vi "Kinesis-Teste-Vector-1.vi"() -> ()   [LabVIEW 2014]
doc: "André Romero - 2017\nandretec@ifsc.usp.br"
uses:
  Basic-VIs/motorsGlobalVar.vi
  <vilib>/Instr/_visa.llb/VISA Configure Serial Port (Instr).vi
  C:/user-Lab/AndreTec/GITs/andretec/Thorlabs-Vector-Move/kinesisTec/Kinesis/Thorlabs.MotionControl.TCube.DCServoCLI.dll
  kinesisTec/Kinesis/Thorlabs.MotionControl.TCube.DCServoCLI.dll
  C:/user-Lab/AndreTec/GITs/andretec/Thorlabs-Vector-Move/kinesisTec/Kinesis/Thorlabs.MotionControl.GenericMotorCLI.dll
  kinesisTec/Kinesis/Thorlabs.MotionControl.GenericMotorCLI.dll
  C:/user-Lab/AndreTec/GITs/andretec/Thorlabs-Vector-Move/kinesisTec/Kinesis/Thorlabs.MotionControl.Controls.dll
  kinesisTec/Kinesis/Thorlabs.MotionControl.Controls.dll
panel:
  out "IsAtHWLimit 2":bool
  out "IsAtHWLimit":bool
  in  "stop":bool
  in  "Adjust Motors":bool
  out "Process time":string="0:00:50"
  out "Progress %":dbl(slide) scale=0.0..100.0
  out "XY Graph":cluster{"Graph X":dbl[], "Graph Y":dbl[]}(graph)
  in  "Swap XY":bool
  out "stop cronometro":bool=TRUE
  in  "Stop Button":bool
  in  "Graph Y":dbl[](array[numeric])=[0.0, 0.0, 6.6674440298507465, 6.6674440298507465, 6.6674440298507465, 6.6674440298507465, 6.6674440298507465, 6.6674440298507465, 6.6674440298507465, 6.6674440298507465, 6.6674440298507465, 6.6674440298507465, 6.6674440298507465, 6.6674440298507465, 6.6674440298507465, 6.6674440298507465, 6.6674440298507465, 6.6674440298507465, 6.6674440298507465, 6.6674440298507465, 6.6674440298507465, 6.6674440298507465, 6.6674440298507465, 6.6674440298507465, 6.6674440298507465, 6.6674440298507465, 6.6674440298507465, 6.6674440298507465, 6.6674440298507465, 6.6674440298507465, 6.6674440298507465, 6.6674440298507465, 6.6674440298507465, 6.6674440298507465, 6.6674440298507465, 6.6674440298507465, 6.6674440298507465, 6.6674440298507465, 6.6674440298507465, 6.6674440298507465, 6.6674440298507465, 6.6674440298507465, 6.6674440298507465, 6.673128498134329, 6.673128498134329, 6.673128498134329, 6.673128498134329, 6.673128498134329, 6.687354244402985, 6.687354244402985, 6.687354244402985, 6.687354244402985, 6.687354244402985, 6.692543143656716, 6.692543143656716, 6.692543143656716, 6.692543143656716, 6.692543143656716, 6.692543143656716, 6.692543143656716, 6.692543143656716, 6.692543143656716, 6.692543143656716, 6.692543143656716, 6.692543143656716, 6.691522854477612, 6.691522854477612, 6.691522854477612, 6.691522854477612, 6.691522854477612, 6.680183069029851, 6.680183069029851, 6.680183069029851, 6.680183069029851, 6.680183069029851, 6.658640391791045, 6.658640391791045, 6.658640391791045, 6.658640391791045, 6.658640391791045, 6.644793610074627, 6.644793610074627, 6.644793610074627, 6.644793610074627, 6.644793610074627, 6.642490671641791, 6.642490671641791, 6.642490671641791, 6.642490671641791, 6.642490671641791, 6.642490671641791, 6.642490671641791, 6.642490671641791, 6.642490671641791, 6.642490671641791, 6.642490671641791, 6.642490671641791, 6.642490671641791, 6.642490671641791, 6.642490671641791, 6.647825326492537, 6.647825326492537, 6.647825326492537, 6.647825326492537, 6.647825326492537, 6.66543260261194, 6.66543260261194, 6.66543260261194, 6.66543260261194, 6.66543260261194, 6.685226212686567, 6.685226212686567, 6.685226212686567, 6.685226212686567, 6.685226212686567, 6.692484841417911, 6.692484841417911, 6.692484841417911, 6.692484841417911, 6.692484841417911, 6.692543143656716, 6.692543143656716, 6.692543143656716, 6.692543143656716, 6.692543143656716, 6.692543143656716, 6.692543143656716, 6.691464552238806, 6.691464552238806, 6.691464552238806, 6.691464552238806, 6.691464552238806, 6.679833255597015, 6.679833255597015, 6.679833255597015, 6.679833255597015, 6.679833255597015, 6.658057369402985, 6.658057369402985, 6.658057369402985, 6.658057369402985, 6.658057369402985, 6.644647854477612, 6.644647854477612, 6.644647854477612, 6.644647854477612, 6.644647854477612, 6.642548973880597, 6.642548973880597, 6.642548973880597, 6.642548973880597, 6.642548973880597, 6.642519822761194, 6.642519822761194, 6.642519822761194, 6.642519822761194, 6.642519822761194, 6.642519822761194, 6.642519822761194, 6.642519822761194, 6.643569263059701, 6.643569263059701, 6.643569263059701, 6.643569263059701, 6.643569263059701, 6.655521222014926, 6.655521222014926, 6.655521222014926, 6.655521222014926, 6.655521222014926, 6.677180503731344, 6.677180503731344, 6.677180503731344, 6.677180503731344, 6.677180503731344, 6.690531716417911, 6.690531716417911, 6.690531716417911, 6.690531716417911, 6.690531716417911, 6.692572294776119, 6.692572294776119, 6.692572294776119, 6.692572294776119, 6.692572294776119, 6.692572294776119, 6.692572294776119, 6.692572294776119, 6.692572294776119, 6.692572294776119, 6.692572294776119, 6.692572294776119, 6.691522854477612, 6.691522854477612, 6.691522854477612, 6.691522854477612, 6.691522854477612, 6.680008162313433, 6.680008162313433, 6.680008162313433, 6.680008162313433, 6.680008162313433, 6.668668376865671, 6.668668376865671, 6.668668376865671, 6.668668376865671, 6.668668376865671, 6.667502332089552, 6.667502332089552, 6.667502332089552, 6.667502332089552, 6.667502332089552, 6.667502332089552, 6.667502332089552, 6.667502332089552, 6.667502332089552, 6.667502332089552, 6.667502332089552, 6.667502332089552, 6.667531483208955, 6.667531483208955, 6.667531483208955, 6.667531483208955, 6.667531483208955, 6.667531483208955, 6.667531483208955, 6.667531483208955, 6.667531483208955, 6.667531483208955, 6.667531483208955, 6.667531483208955, 6.667531483208955, 6.667531483208955, 6.667531483208955, 6.667531483208955, 6.667531483208955, 6.667531483208955, 6.667531483208955, 6.667531483208955, 6.667531483208955, 6.667531483208955, 6.667531483208955, 6.667531483208955, 6.667531483208955, 6.667531483208955, 6.667531483208955, 6.667531483208955, 6.667531483208955, 6.667531483208955, 6.667531483208955, 6.667531483208955, 6.667531483208955, 6.667531483208955, 6.667531483208955, 6.667531483208955, 6.667531483208955, 6.6663945895522385, 6.6663945895522385, 6.6663945895522385, 6.6663945895522385, 6.6663945895522385, 6.662051072761194, 6.662051072761194, 6.662051072761194, 6.662051072761194, 6.662051072761194, 6.644035680970149, 6.644035680970149, 6.644035680970149, 6.644035680970149, 6.644035680970149, 6.606430736940299, 6.606430736940299, 6.606430736940299, 6.606430736940299, 6.606430736940299, 6.593924906716418, 6.593924906716418, 6.593924906716418, 6.593924906716418, 6.593924906716418, 6.574539412313433, 6.574539412313433, 6.574539412313433, 6.574539412313433, 6.574539412313433, 6.567484841417911, 6.567484841417911, 6.567484841417911, 6.567484841417911, 6.567484841417911, 6.567484841417911, 6.567484841417911, 6.567484841417911, 6.567484841417911, 6.567484841417911, 6.567484841417911, 6.567513992537314, 6.567513992537314, 6.567513992537314, 6.567513992537314, 6.567513992537314, 6.567513992537314, 6.567513992537314, 6.567513992537314, 6.567513992537314, 6.567513992537314, 6.567543143656716, 6.567543143656716, 6.567543143656716, 6.567543143656716, 6.567543143656716, 6.567543143656716, 6.567543143656716, 6.567543143656716, 6.567543143656716, 6.567543143656716, 6.567543143656716, 6.567543143656716, 6.567543143656716, 6.567543143656716, 6.567543143656716, 6.567543143656716, 6.567543143656716, 6.567543143656716, 6.567543143656716, 6.567543143656716, 6.567543143656716, 6.567543143656716, 6.567543143656716, 6.567543143656716, 6.567543143656716, 6.567543143656716, 6.567543143656716, 6.567543143656716, 6.567543143656716, 6.567543143656716, 6.567543143656716, 6.567543143656716, 6.567543143656716, 6.567543143656716, 6.567543143656716, 6.567543143656716, 6.567543143656716, 6.567543143656716, 6.567543143656716, 6.567543143656716, 6.567543143656716, 6.567543143656716, 6.567543143656716, 6.567543143656716, 6.567543143656716, 6.567543143656716, 6.567543143656716, 6.567543143656716, 6.567543143656716, 6.567543143656716, 6.567543143656716, 6.567543143656716, 6.567543143656716, 6.567543143656716, 6.5667852145522385, 6.5667852145522385, 6.5667852145522385, 6.5667852145522385, 6.5667852145522385, 6.555299673507463, 6.555299673507463, 6.555299673507463, 6.555299673507463, 6.555299673507463, 6.533523787313433, 6.533523787313433, 6.533523787313433, 6.533523787313433, 6.533523787313433, 6.525186567164179, 6.525186567164179, 6.525186567164179, 6.525186567164179, 6.525186567164179, 6.517490671641791, 6.517490671641791, 6.517490671641791, 6.517490671641791, 6.517490671641791, 6.517490671641791, 6.517490671641791, 6.517490671641791, 6.517490671641791, 6.517490671641791, 6.517519822761194, 6.517519822761194, 6.517519822761194, 6.517519822761194, 6.517519822761194, 6.517519822761194, 6.517519822761194, 6.517519822761194, 6.517519822761194, 6.517519822761194, 6.517548973880597, 6.517548973880597, 6.517548973880597, 6.517548973880597, 6.517548973880597, 6.517548973880597, 6.517548973880597, 6.517548973880597, 6.517548973880597, 6.517548973880597, 6.517548973880597, 6.517548973880597, 6.517548973880597, 6.517548973880597, 6.517548973880597, 6.517548973880597, 6.517548973880597, 6.517548973880597, 6.517548973880597, 6.517548973880597, 6.517548973880597, 6.517548973880597, 6.517548973880597, 6.517548973880597, 6.517548973880597, 6.517548973880597, 6.517548973880597, 6.517548973880597, 6.517548973880597, 6.517548973880597, 6.517548973880597, 6.517548973880597, 6.517548973880597, 6.517548973880597, 6.517548973880597, 6.517548973880597, 6.517548973880597, 6.517548973880597, 6.517548973880597, 6.517548973880597, 6.517548973880597, 6.517548973880597, 6.517548973880597, 6.517548973880597, 6.517548973880597, 6.517548973880597, 6.517548973880597, 6.517548973880597, 6.517548973880597, 6.517548973880597, 6.517548973880597, 6.517548973880597, 6.517548973880597, 6.517548973880597, 6.517548973880597, 6.517548973880597, 6.517548973880597, 6.517548973880597, 6.517548973880597, 6.517548973880597, 6.516674440298507, 6.516674440298507, 6.516674440298507, 6.516674440298507, 6.516674440298507, 6.504897388059701, 6.504897388059701, 6.504897388059701, 6.504897388059701, 6.504897388059701, 6.481926305970149, 6.481926305970149, 6.481926305970149, 6.481926305970149, 6.481926305970149, 6.456943796641791, 6.456943796641791, 6.456943796641791, 6.456943796641791, 6.456943796641791, 6.4330690298507465, 6.4330690298507465, 6.4330690298507465, 6.4330690298507465, 6.4330690298507465, 6.419717817164179, 6.419717817164179, 6.419717817164179, 6.419717817164179, 6.419717817164179, 6.417473180970149, 6.417473180970149, 6.417473180970149, 6.417473180970149, 6.417473180970149, 6.417473180970149]
  in  "Graph X":dbl[](array[numeric])=[0.0, 0.0, 3.605935167910448, 3.605935167910448, 3.605935167910448, 3.605935167910448, 3.605935167910448, 3.609987173507463, 3.609987173507463, 3.609987173507463, 3.609987173507463, 3.609987173507463, 3.627157182835821, 3.627157182835821, 3.627157182835821, 3.627157182835821, 3.627157182835821, 3.6520813899253732, 3.6520813899253732, 3.6520813899253732, 3.6520813899253732, 3.6520813899253732, 3.6770930503731343, 3.6770930503731343, 3.6770930503731343, 3.6770930503731343, 3.6770930503731343, 3.697323927238806, 3.697323927238806, 3.697323927238806, 3.697323927238806, 3.697323927238806, 3.705311333955224, 3.705311333955224, 3.705311333955224, 3.705311333955224, 3.705311333955224, 3.705311333955224, 3.705311333955224, 3.705311333955224, 3.705311333955224, 3.705311333955224, 3.705311333955224, 3.7063024720149254, 3.7063024720149254, 3.7063024720149254, 3.7063024720149254, 3.7063024720149254, 3.7175839552238807, 3.7175839552238807, 3.7175839552238807, 3.7175839552238807, 3.7175839552238807, 3.7291861007462686, 3.7291861007462686, 3.7291861007462686, 3.7291861007462686, 3.7291861007462686, 3.7303521455223883, 3.7303521455223883, 3.7303521455223883, 3.7303521455223883, 3.7303521455223883, 3.7303521455223883, 3.7303521455223883, 3.7303521455223883, 3.7303521455223883, 3.7303521455223883, 3.7303521455223883, 3.7303521455223883, 3.7366779384328357, 3.7366779384328357, 3.7366779384328357, 3.7366779384328357, 3.7366779384328357, 3.7554221082089554, 3.7554221082089554, 3.7554221082089554, 3.7554221082089554, 3.7554221082089554, 3.774137126865672, 3.774137126865672, 3.774137126865672, 3.774137126865672, 3.774137126865672, 3.7803463152985075, 3.7803463152985075, 3.7803463152985075, 3.7803463152985075, 3.7803463152985075, 3.7803463152985075, 3.7803463152985075, 3.7803463152985075, 3.7803463152985075, 3.7803463152985075, 3.7803463152985075, 3.7803463152985075, 3.7803463152985075, 3.7803463152985075, 3.7803463152985075, 3.781803871268657, 3.781803871268657, 3.781803871268657, 3.781803871268657, 3.781803871268657, 3.7941930970149254, 3.7941930970149254, 3.7941930970149254, 3.7941930970149254, 3.7941930970149254, 3.816027285447761, 3.816027285447761, 3.816027285447761, 3.816027285447761, 3.816027285447761, 3.828678871268657, 3.828678871268657, 3.828678871268657, 3.828678871268657, 3.828678871268657, 3.8303404850746268, 3.8303404850746268, 3.8303404850746268, 3.8303404850746268, 3.8303404850746268, 3.8303404850746268, 3.8303404850746268, 3.8303404850746268, 3.8303404850746268, 3.8303404850746268, 3.8303404850746268, 3.8303404850746268, 3.8368703358208953, 3.8368703358208953, 3.8368703358208953, 3.8368703358208953, 3.8368703358208953, 3.8447994402985075, 3.8447994402985075, 3.8447994402985075, 3.8447994402985075, 3.8447994402985075, 3.866633628731343, 3.866633628731343, 3.866633628731343, 3.866633628731343, 3.866633628731343, 3.8803346548507465, 3.8803346548507465, 3.8803346548507465, 3.8803346548507465, 3.8803346548507465, 3.8803346548507465, 3.8803346548507465, 3.8803346548507465, 3.8803346548507465, 3.8803346548507465, 3.8803346548507465, 3.8803346548507465, 3.8803346548507465, 3.8803346548507465, 3.8803346548507465, 3.8803346548507465, 3.8803346548507465, 3.8803346548507465, 3.886631296641791, 3.886631296641791, 3.886631296641791, 3.886631296641791, 3.886631296641791, 3.9054046175373136, 3.9054046175373136, 3.9054046175373136, 3.9054046175373136, 3.9054046175373136, 3.92411963619403, 3.92411963619403, 3.92411963619403, 3.92411963619403, 3.92411963619403, 3.9303288246268657, 3.9303288246268657, 3.9303288246268657, 3.9303288246268657, 3.9303288246268657, 3.9303288246268657, 3.9303288246268657, 3.9303288246268657, 3.9303288246268657, 3.9303288246268657, 3.9303288246268657, 3.9303288246268657, 3.9303288246268657, 3.9303288246268657, 3.9303288246268657, 3.9303288246268657, 3.9303288246268657, 3.936800373134328, 3.936800373134328, 3.936800373134328, 3.936800373134328, 3.936800373134328, 3.9445545708955225, 3.9445545708955225, 3.9445545708955225, 3.9445545708955225, 3.9445545708955225, 3.95536963619403, 3.95536963619403, 3.95536963619403, 3.95536963619403, 3.95536963619403, 3.95536963619403, 3.95536963619403, 3.95536963619403, 3.95536963619403, 3.95536963619403, 3.95536963619403, 3.95536963619403, 3.956652285447761, 3.956652285447761, 3.956652285447761, 3.956652285447761, 3.956652285447761, 3.961141557835821, 3.961141557835821, 3.961141557835821, 3.961141557835821, 3.961141557835821, 3.9795067630597014, 3.9795067630597014, 3.9795067630597014, 3.9795067630597014, 3.9795067630597014, 4.004518423507463, 4.004518423507463, 4.004518423507463, 4.004518423507463, 4.004518423507463, 4.0406366604477615, 4.0406366604477615, 4.0406366604477615, 4.0406366604477615, 4.0406366604477615, 4.048624067164179, 4.048624067164179, 4.048624067164179, 4.048624067164179, 4.048624067164179, 4.0553579757462686, 4.0553579757462686, 4.0553579757462686, 4.0553579757462686, 4.0553579757462686, 4.0553579757462686, 4.0553579757462686, 4.055387126865671, 4.055387126865671, 4.055387126865671, 4.055387126865671, 4.055387126865671, 4.055387126865671, 4.055387126865671, 4.055387126865671, 4.055387126865671, 4.055387126865671, 4.0553579757462686, 4.0553579757462686, 4.0553579757462686, 4.0553579757462686, 4.0553579757462686, 4.0553579757462686, 4.0553579757462686, 4.0553579757462686, 4.0553579757462686, 4.0553579757462686, 4.0553579757462686, 4.0553579757462686, 4.0553579757462686, 4.0553579757462686, 4.0553579757462686, 4.0553579757462686, 4.0553579757462686, 4.0553579757462686, 4.0553579757462686, 4.0553579757462686, 4.0553579757462686, 4.0553579757462686, 4.0553579757462686, 4.0553579757462686, 4.0553579757462686, 4.0553579757462686, 4.0553579757462686, 4.0553579757462686, 4.0553579757462686, 4.0553579757462686, 4.0553579757462686, 4.061800373134329, 4.061800373134329, 4.061800373134329, 4.061800373134329, 4.061800373134329, 4.06972947761194, 4.06972947761194, 4.06972947761194, 4.06972947761194, 4.06972947761194, 4.091534514925373, 4.091534514925373, 4.091534514925373, 4.091534514925373, 4.091534514925373, 4.105352145522388, 4.105352145522388, 4.105352145522388, 4.105352145522388, 4.105352145522388, 4.105381296641791, 4.105381296641791, 4.105381296641791, 4.105381296641791, 4.105381296641791, 4.105381296641791, 4.105381296641791, 4.1050897854477615, 4.1050897854477615, 4.1050897854477615, 4.1050897854477615, 4.1050897854477615, 4.0951784048507465, 4.0951784048507465, 4.0951784048507465, 4.0951784048507465, 4.0951784048507465, 4.073489972014926, 4.073489972014926, 4.073489972014926, 4.073489972014926, 4.073489972014926, 4.060954990671642, 4.060954990671642, 4.060954990671642, 4.060954990671642, 4.060954990671642, 4.023874766791045, 4.023874766791045, 4.023874766791045, 4.023874766791045, 4.023874766791045, 4.008687033582089, 4.008687033582089, 4.008687033582089, 4.008687033582089, 4.008687033582089, 4.005363805970149, 4.005363805970149, 4.005363805970149, 4.005363805970149, 4.005363805970149, 4.005363805970149, 4.005363805970149, 4.005363805970149, 4.005363805970149, 4.005363805970149, 4.005363805970149, 4.005363805970149, 4.005363805970149, 4.005363805970149, 4.005363805970149, 4.005363805970149, 4.005363805970149, 4.005392957089552, 4.005392957089552, 4.005392957089552, 4.005392957089552, 4.005392957089552, 4.005392957089552, 4.005392957089552, 4.005392957089552, 4.005392957089552, 4.005392957089552, 4.005392957089552, 4.005392957089552, 4.005392957089552, 4.005392957089552, 4.005392957089552, 4.005392957089552, 4.005392957089552, 4.005392957089552, 4.005392957089552, 4.005392957089552, 4.011631296641791, 4.011631296641791, 4.011631296641791, 4.011631296641791, 4.011631296641791, 4.019472947761194, 4.019472947761194, 4.019472947761194, 4.019472947761194, 4.019472947761194, 4.042852145522388, 4.042852145522388, 4.042852145522388, 4.042852145522388, 4.042852145522388, 4.080398787313433, 4.080398787313433, 4.080398787313433, 4.080398787313433, 4.080398787313433, 4.099113805970149, 4.099113805970149, 4.099113805970149, 4.099113805970149, 4.099113805970149, 4.103777985074627, 4.103777985074627, 4.103777985074627, 4.103777985074627, 4.103777985074627, 4.105410447761194, 4.105410447761194, 4.105410447761194, 4.105410447761194, 4.105410447761194, 4.105410447761194, 4.105410447761194, 4.105410447761194, 4.105381296641791, 4.105381296641791, 4.105381296641791, 4.105381296641791, 4.105381296641791, 4.098297574626866, 4.098297574626866, 4.098297574626866, 4.098297574626866, 4.098297574626866, 4.089989505597015, 4.089989505597015, 4.089989505597015, 4.089989505597015, 4.089989505597015, 4.06083838619403, 4.06083838619403, 4.06083838619403, 4.06083838619403, 4.06083838619403, 4.0553579757462686, 4.0553579757462686, 4.0553579757462686, 4.0553579757462686, 4.0553579757462686, 4.0553579757462686, 4.0553579757462686, 4.0553579757462686, 4.0553579757462686, 4.0553579757462686, 4.0553579757462686, 4.0553579757462686, 4.055387126865671, 4.055387126865671, 4.055387126865671, 4.055387126865671, 4.055387126865671, 4.055416277985074, 4.055416277985074, 4.055416277985074, 4.055416277985074, 4.055416277985074, 4.055416277985074, 4.055416277985074, 4.055416277985074, 4.055416277985074, 4.055416277985074, 4.055416277985074, 4.055416277985074, 4.055416277985074, 4.055416277985074, 4.055416277985074, 4.055416277985074, 4.055416277985074, 4.055416277985074, 4.055416277985074, 4.055416277985074, 4.055416277985074, 4.055416277985074, 4.055416277985074, 4.055416277985074, 4.055416277985074, 4.055416277985074, 4.055416277985074, 4.055416277985074, 4.055416277985074, 4.055416277985074, 4.055416277985074]
  out "GetPOS Y":dbl=6.417473180970149 format="%_6f"
  out "GetPOS X":dbl=4.055416277985074 format="%#_6f"
  out ".NET Refnum out 2":refnum<k24>
  out ".NET Refnum out 1":refnum<k24>
  out "Motor 2":bool
  out "Motor 1":bool
  in  "Acceleration (mm/s)":dbl=0.05
  in  "Iniciar":bool
  in  "Velocity (mm/s)":sgl=0.05
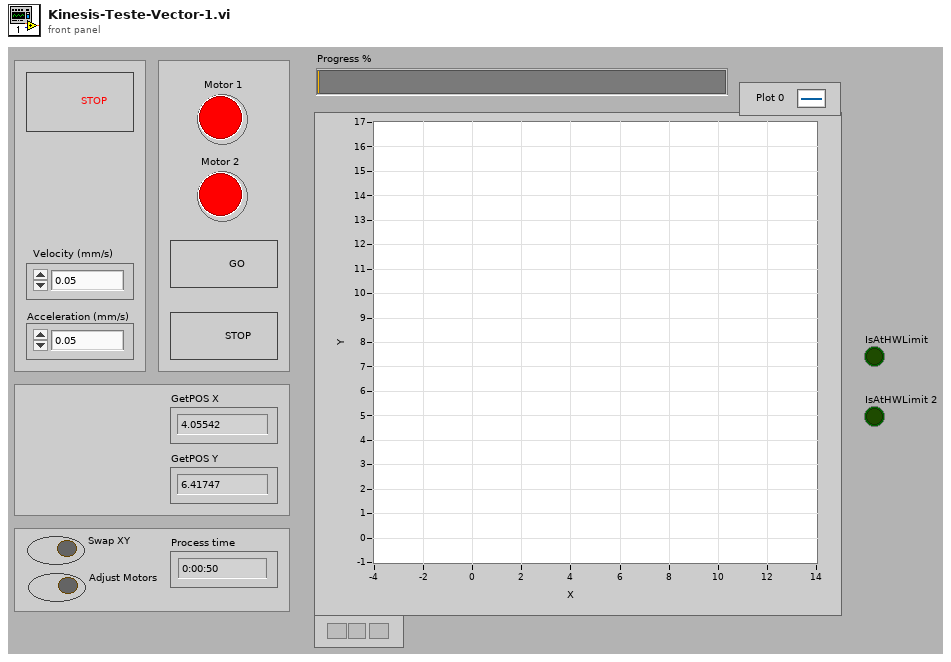
[diagram p1: front panel]
types:
  T1 = enum8{"Enabled", "Disabled", "Disabled and Grayed Out"}
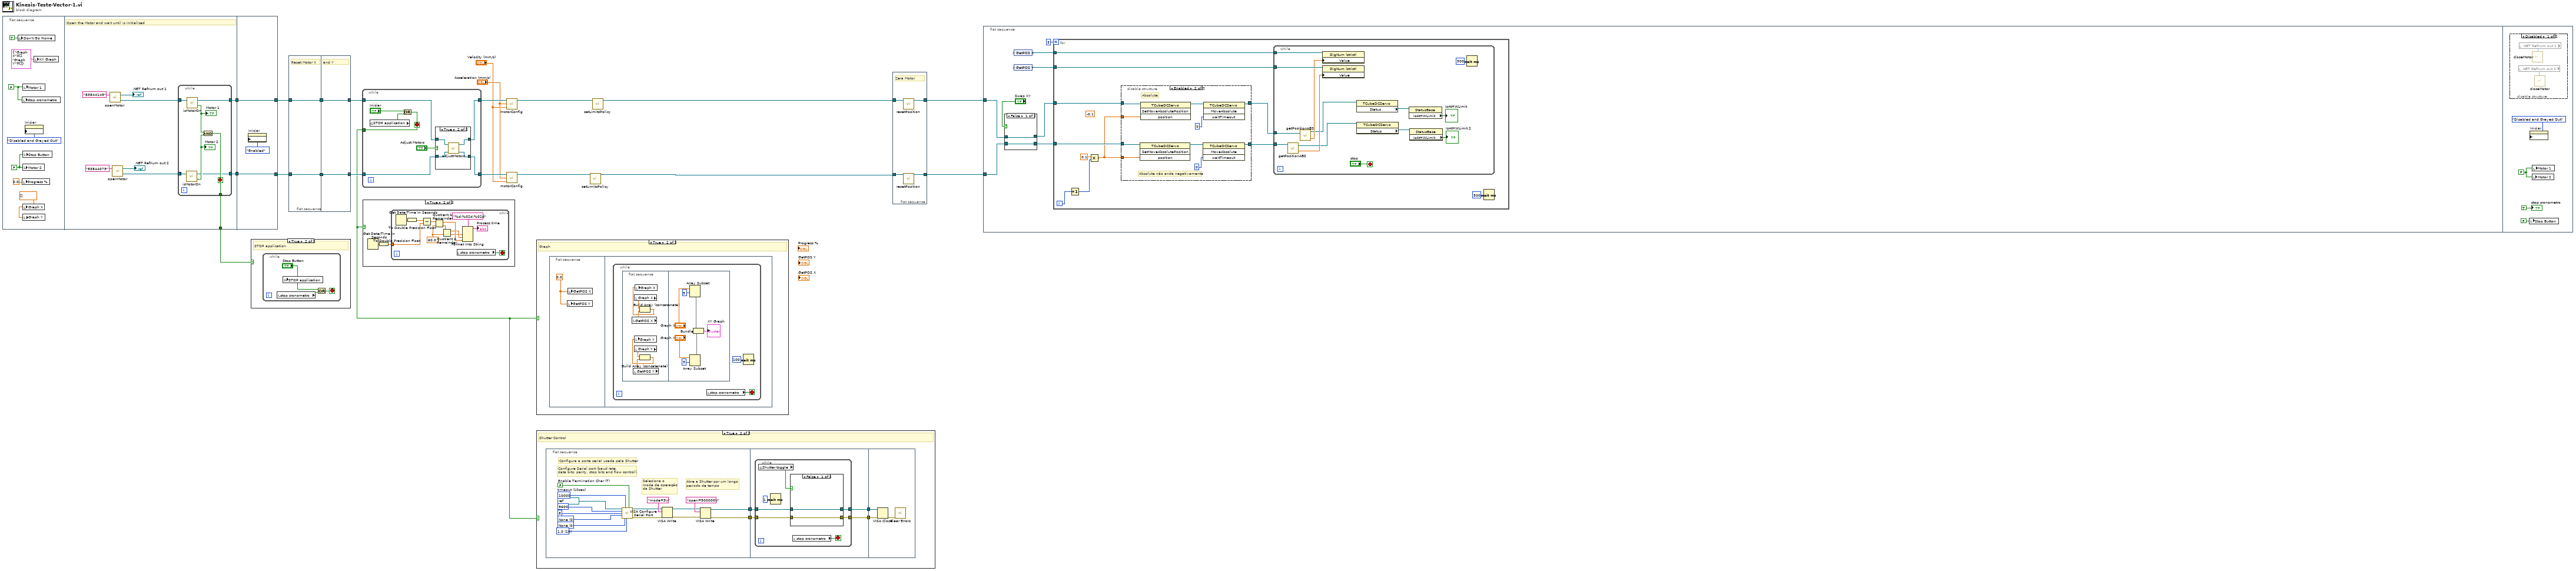
[diagram p0: block diagram]
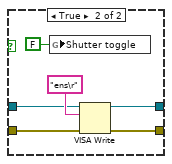
[diagram p3: hidden frame]
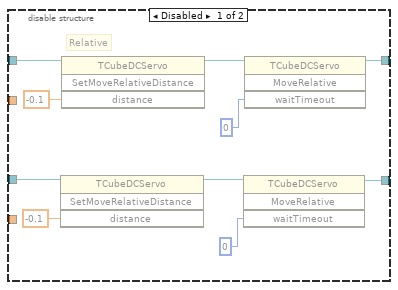
[diagram p6: hidden frame]
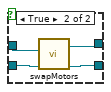
[diagram p7: hidden frame]
diagram:
  n1 = flat-sequence {
    tunnel: [w36] -> w10
    tunnel: [w35] -> w9
    tunnel: [w34] -> w8
    tunnel: [w45] -> w13
    tunnel: [w46] -> w14
    tunnel: w10 -> [w46]
    tunnel: w9 -> [w45]
    frame #0 {
      w23 = dbl[] [] ("Graph Y")
      w26 = FALSE ("Motor3\nLigado")
      w27 = FALSE
      n2 = global write "motorsGlobalVar.vi" "Don't Go Home"(TRUE ("Don't Go Home")) -> ()
      n3 = local write "stop cronometro"(w27) -> ()
      n4 = local write "Progress %"(0.0 ("Progress %")) -> ()
      n5 = local write "Motor 2"(w26) -> ()
      n6 = local write "Graph X"(w23) -> ()
      n7 = local write "Motor 1"(w27) -> ()
      n8 = local write "Stop Button"(w26) -> ()
      n9 = local write "Graph Y"(w23) -> ()
      n10 = property on="Iniciar" class="Bool (strict)"("DisabledEnum"=T1."Disabled and Grayed Out" ("Disabled")) -> ()  [unwired: 2 in, 2 out]
      n11 = local write "XY Graph"(cluster{"Graph X":dbl[], "Graph Y":dbl[]} {"Graph X"=[], "Graph Y"=[]} ("XY Graph")) -> ()
    }
    frame #1 {
      # "Open the Motor and wait until is initialized"
      n12 = call "openMotor.vi"("S/N Motor"="83844149") -> ("Device"=w32:refnum<k24>, ".NET Refnum out"=→".NET Refnum out 1":refnum<k24>)  [unwired: 1 in]
      n13 = call "openMotor.vi"("S/N Motor"="83844079") -> ("Device"=w33:refnum<k24>, ".NET Refnum out"=→".NET Refnum out 2":refnum<k24>)  [unwired: 1 in]
      n14 = while {
        tunnel: w32 -> [w41]
        tunnel: w33 -> [w40]
        tunnel: [w38] -> w36
        tunnel: [w37] -> w35
        tunnel: [w39] -> w34
        stop <- w39 stop-if-true
        n15 = call "isMotorOn.vi"("Device"=w40) -> ("isConnected"=w42:bool, "Device out"=w37:refnum<k24>)  [unwired: 1 in]
        "Motor 2" <- w42
        n16 = call "isMotorOn.vi"("Device"=w41) -> ("isConnected"=w43:bool, "Device out"=w38:refnum<k24>)  [unwired: 1 in]
        "Motor 1" <- w43
        n17 = And(x=w43, y=w42) -> (x .and. y?=w39:bool)
      }
    }
    frame #2 {
      n18 = property on="Iniciar" class="Bool (strict)"("DisabledEnum"=T1."Enabled" ("Disabled")) -> ()  [unwired: 2 in, 2 out]
    }
  }
  n19 = case shown="True" w8 {
    frame False {
    }
    frame True {
      # "STOP application"
      n20 = while {
        stop <- w48 stop-if-true
        n21 = local read "stop cronometro"() -> (w47:bool)
        n22 = global write "motorsGlobalVar.vi" "STOP application"("Stop Button") -> ()
        n23 = Or(x="Stop Button", y=w47) -> (x .or. y?=w48:bool)
      }
    }
  }
  n24 = flat-sequence {
    tunnel: w14 -> [w50]
    tunnel: w13 -> [w51]
    tunnel: [w50] -> w12
    tunnel: [w51] -> w11
    tunnel: [w53] -> w16
    tunnel: [w52] -> w15
    tunnel: w12 -> [w53]
    tunnel: w11 -> [w52]
    frame #0 {
      # "Reset Motor X"
    }
    frame #1 {
      # "and Y"
    }
  }
  n25 = while {
    tunnel: [w61] -> w7
    tunnel: w16 -> [w56]
    tunnel: w15 -> [w57]
    tunnel: [w55] -> w20
    tunnel: [w54] -> w19
    stop <- w61 stop-if-true
    n26 = global read "motorsGlobalVar.vi" "STOP application"() -> (w59:bool)
    n27 = Or(x="Iniciar", y=w59) -> (x .or. y?=w61:bool)
    n28 = case shown="True" "Adjust Motors" {
      tunnel: w57 -> [w62 w67]
      tunnel: w56 -> [w63 w66]
      tunnel: [w63 w65] -> w55
      tunnel: [w62 w64] -> w54
      frame False {
      }
      frame True {
        n29 = call "adjustMotors.vi"("Device 2"=w67, "Device 1"=w66) -> ("Device out 2"=w64:refnum<k24>, "Device out 1"=w65:refnum<k24>)  [unwired: 2 in]
      }
    }
  }
  n30 = case shown="True" w7 {
    frame False {
    }
    frame True {
      n31 = Get Date/Time In Seconds() -> (seconds since 1Jan1904=w69:timestamp)
      n32 = To Double Precision Float(number=w69) -> (double precision float=w68:dbl)
      n33 = while {
        tunnel: w68 -> [w73]
        stop <- w81 stop-if-true
        w78 = 60.0 ("y")
        n34 = Get Date/Time In Seconds() -> (seconds since 1Jan1904=w80:timestamp)
        n35 = To Double Precision Float(number=w80) -> (double precision float=w74:dbl)
        n36 = Subtract(x=w74, y=w73) -> (x-y=w72:dbl)
        n37 = Quotient & Remainder(x=w72, y=w78) -> (x-y*floor(x/y)=w77:dbl, floor(x/y)=w79:dbl)
        n38 = Quotient & Remainder(x=w79, y=w78) -> (x-y*floor(x/y)=w76:dbl, floor(x/y)=w75:dbl)
        n39 = local read "stop cronometro"() -> (w81:bool)
        n40 = Format Into String(format string="%d:%02d:%02d", w75, w76, w77) -> (resulting string=→"Process time":string)  [unwired: 2 in, 1 out]
      }
    }
  }
  n41 = call "motorConfig.vi"("Velocity"="Velocity (mm/s)", "Acceleration"="Acceleration (mm/s)", "Device in"=w20) -> ("Device out"=w4:refnum<k24>)  [unwired: 2 in]
  n42 = call "motorConfig.vi"("Velocity"="Velocity (mm/s)", "Acceleration"="Acceleration (mm/s)", "Device in"=w19) -> ("Device out"=w2:refnum<k24>)  [unwired: 2 in]
  n43 = case shown="True" w7 {
    frame False {
    }
    frame True {
      # "Graph"
      n44 = flat-sequence {
        frame #0 {
          w82 = 0.0
          n45 = local write "GetPOS Y"(w82) -> ()
          n46 = local write "GetPOS X"(w82) -> ()
        }
        frame #1 {
          n47 = while {
            stop <- w83 stop-if-true
            n48 = flat-sequence {
              frame #0 {
                n49 = local read "GetPOS X"() -> (w88:dbl)
                n50 = local read "GetPOS Y"() -> (w87:dbl)
                n51 = local read "Graph X"() -> (w90:dbl[])
                n52 = local read "Graph Y"() -> (w85:dbl[])
                n53 = Build Array (concatenate)(w90, w88) -> (w89:dbl[])
                n54 = local write "Graph X"(w89) -> ()
                n55 = Build Array (concatenate)(w85, w87) -> (w86:dbl[])
                n56 = local write "Graph Y"(w86) -> ()
              }
              frame #1 {
                n57 = Array Subset(array="Graph Y", index=3) -> (w91:dbl[])  [unwired: 1 in]
                n58 = Array Subset(array="Graph X", index=3) -> (w94:dbl[])  [unwired: 1 in]
                n59 = Bundle(w94, w91) -> (→"XY Graph":cluster{dbl[], dbl[]})  [unwired: 1 in]
              }
            }
            n60 = local read "stop cronometro"() -> (w83:bool)
            n61 = Wait (ms)(milliseconds to wait=u32 100) -> ()  [unwired: 1 out]
          }
        }
      }
    }
  }
  n62 = case shown="True" w7 {
    frame False {
    }
    frame True {
      # "Shutter Control"
      n63 = flat-sequence {
        tunnel: [w103] -> w101
        tunnel: [w102] -> w100
        tunnel: w101 -> [w121]
        tunnel: w100 -> [w118]
        tunnel: [w120] -> w99
        tunnel: [w119] -> w98
        tunnel: w99 -> [w139]
        tunnel: w98 -> [w138]
        frame #0 {
          w113 = u16 0 items=["None", "Odd", "Even", "Mark", "Space"] ("parity")
          w110 = u16 10 items=["1.0"=10, "1.5"=15, "2.0"=20] ("stop bits")
          w109 = u16 0 items=["None"=0, "XON/XOFF"=1, "RTS/CTS"=2, "DTR/DSR"=4] ("flow control")
          w111 = FALSE  # Enable Termination Char (T)
          w112 = u32 10000  # timeout (10sec)
          # "Configura a porta serial usada pela Shutter"
          # "Configure Serial port (baud rate,\ndata bits, parity, stop bits and flow control)."
          # "Seleciona o \nmode de operação\nda Shutter"
          # "Abre a Shutter por um longo\nperíodo de tempo"
          n64 = call-poly "VISA Configure Serial Port"("VISA resource name"=refnum<visa-resource-name> "COM3", "timeout (10sec)"=w112, "Enable Termination\nChar (T)"=w111, "baud rate (9600)"=u32 9600 ("baud rate"), "data bits (8)"=u16 8 ("data bits"), "parity (0:none)"=w113, "stop bits (10: 1 bit)"=w110, "flow control (0:none)"=w109) -> ("VISA resource name out"=w107:refnum<visa-resource-name>, "error out"=w106:errorcluster)  [unwired: 6 in]
          n65 = VISA Write(VISA resource name=w107, write buffer="mode=3\r", error in (no error)=w106) -> (VISA resource name out=w105:refnum<visa-resource-name>, error out=w104:errorcluster)  [unwired: 1 out]
          n66 = VISA Write(VISA resource name=w105, write buffer="open=900000\r", error in (no error)=w104) -> (VISA resource name out=w103:refnum<visa-resource-name>, error out=w102:errorcluster)  [unwired: 1 out]
        }
        frame #1 {
          n67 = while {
            tunnel: w121 -> [w128]
            tunnel: [w127] -> w120
            tunnel: [w126] -> w119
            tunnel: w118 -> [w125]
            stop <- w122 stop-if-true
            n68 = global read "motorsGlobalVar.vi" "Shutter toggle"() -> (w124:bool)
            n69 = Wait (ms)(milliseconds to wait=u32 1) -> ()  [unwired: 1 out]
            n70 = case shown="False" w124 {
              tunnel: w128 -> [w130 w135]
              tunnel: [w130 w134] -> w127
              tunnel: [w129 w133] -> w126
              tunnel: w125 -> [w129 w132]
              frame False {
              }
              frame True {
                n71 = global write "motorsGlobalVar.vi" "Shutter toggle"(FALSE ("Shutter toggle")) -> ()
                n72 = VISA Write(VISA resource name=w135, write buffer="ens\r", error in (no error)=w132) -> (VISA resource name out=w134:refnum<visa-resource-name>, error out=w133:errorcluster)  [unwired: 1 out]
              }
            }
            n73 = local read "stop cronometro"() -> (w122:bool)
          }
        }
        frame #2 {
          n74 = VISA Close(VISA resource name=w139, error in (no error)=w138) -> (error out=w137:errorcluster)
          n75 = call <vilib>:"Clear Errors.vi"("error in (no error)"=w137) -> ()  [unwired: 5 in, 2 out]
        }
      }
    }
  }
  n76 = call "setLimitsPolicy.vi"("Device in"=w2) -> ("Device out"=w1:refnum<k24>)  [unwired: 10 in]
  n77 = call "setLimitsPolicy.vi"("Device in"=w4) -> ("Device out"=w3:refnum<k24>)  [unwired: 10 in]
  n78 = flat-sequence {
    tunnel: w3 -> [w143]
    tunnel: w1 -> [w141]
    tunnel: [w142] -> w6
    tunnel: [w140] -> w5
    frame #0 {
      # "Zera Motor"
      n79 = call "resetPosition.vi"("Device in"=w143) -> ("Device out"=w142:refnum<k24>)  [unwired: 10 in]
      n80 = call "resetPosition.vi"("Device in"=w141) -> ("Device out"=w140:refnum<k24>)  [unwired: 10 in]
    }
  }
  n81 = flat-sequence {
    tunnel: w6 -> [w151]
    tunnel: w5 -> [w150]
    frame #0 {
      n82 = case shown="False" "Swap XY" {
        tunnel: w151 -> [w198 w202]
        tunnel: w150 -> [w197 w201]
        tunnel: [w198 w200] -> w146
        tunnel: [w197 w199] -> w145
        frame False {
        }
        frame True {
          n83 = call "swapMotors.vi"("Device 2"=w201, "Device 1"=w202) -> ("Device out 1"=w199:refnum<k24>, "Device out 2"=w200:refnum<k24>)  [unwired: 2 in, 2 out]
        }
      }
      n84 = control-ref of="GetPOS X"() -> (w148:refnum<vi>)
      n85 = control-ref of="GetPOS Y"() -> (w147:refnum<vi>)
      n86 = for {
        N: 3 -> [_]
        tunnel: w148 -> [w162]
        tunnel: w147 -> [w161]
        tunnel: w146 -> [w160]
        tunnel: w145 -> [w159]
        i -> [w154]
        (unwired) -0.1 ("position")
        n87 = Increment(x=w154) -> (x+1=w153:i32)
        n88 = Multiply(x=0.1 ("position"), y=w153) -> (x*y=w152:dbl)
        n89 = disable-structure shown="Enabled" {
          disable-tunnel: w160 -> [w170 w178]
          disable-tunnel: w159 -> [w165 w177]
          disable-tunnel: [w164 w175] -> w158
          disable-tunnel: [w163 w176] -> w156
          disable-tunnel: w152 -> [_ w174]
          disable-tunnel: w152 -> [_ w173]
          frame Disabled {
            # "Relative"
            n90 = invoke class="TCubeDCServo" method="SetMoveRelativeDistance"(reference=w165, "distance"=-0.1 ("position")) -> (reference out=w168:refnum<k24>)  [unwired: 2 in, 3 out]
            n91 = invoke class="TCubeDCServo" method="SetMoveRelativeDistance"(reference=w170, "distance"=-0.1 ("position")) -> (reference out=w172:refnum<k24>)  [unwired: 2 in, 3 out]
            n92 = invoke class="TCubeDCServo" method="MoveRelative"(reference=w168, "waitTimeout"=0) -> (reference out=w164:refnum<k24>)  [unwired: 2 in, 3 out]
            n93 = invoke class="TCubeDCServo" method="MoveRelative"(reference=w172, "waitTimeout"=0) -> (reference out=w163:refnum<k24>)  [unwired: 2 in, 3 out]
          }
          frame Enabled {
            # "Absolute não anda negativamente"
            # "Absolute"
            n94 = invoke class="TCubeDCServo" method="SetMoveAbsolutePosition"(reference=w177, "position"=w174) -> (reference out=w180:refnum<k24>)  [unwired: 2 in, 3 out]
            n95 = invoke class="TCubeDCServo" method="SetMoveAbsolutePosition"(reference=w178, "position"=w173) -> (reference out=w182:refnum<k24>)  [unwired: 2 in, 3 out]
            n96 = invoke class="TCubeDCServo" method="MoveAbsolute"(reference=w180, "waitTimeout"=0) -> (reference out=w175:refnum<k24>)  [unwired: 2 in, 3 out]
            n97 = invoke class="TCubeDCServo" method="MoveAbsolute"(reference=w182, "waitTimeout"=0) -> (reference out=w176:refnum<k24>)  [unwired: 2 in, 3 out]
          }
        }
        n98 = while {
          tunnel: w162 -> [w196]
          tunnel: w161 -> [w195]
          tunnel: w156 -> [w192]
          tunnel: w158 -> [w191]
          stop <- "stop" stop-if-true
          n99 = call "getPositionABS.vi"("Device"=w191) -> ("GetPOS"=w193:dbl, "Device out"=w183:refnum<k24>)  [unwired: 1 in]
          n100 = call "getPositionABS.vi"("Device"=w192) -> ("GetPOS"=w194:dbl, "Device out"=w189:refnum<k24>)  [unwired: 1 in]
          n101 = property class="DigNum (strict)"(reference=w196, "Value"=w194) -> ()  [unwired: 1 in, 2 out]
          n102 = property class="DigNum (strict)"(reference=w195, "Value"=w193) -> ()  [unwired: 1 in, 2 out]
          n103 = property class="TCubeDCServo"(reference=w189) -> ("Status"=w188:refnum<k24>)  [unwired: 1 in, 2 out]
          n104 = property class="TCubeDCServo"(reference=w183) -> ("Status"=w186:refnum<k24>)  [unwired: 1 in, 2 out]
          n105 = property class="StatusBase"(reference=w188) -> ("IsAtHWLimit"=→"IsAtHWLimit":bool)  [unwired: 1 in, 2 out]
          n106 = property class="StatusBase"(reference=w186) -> ("IsAtHWLimit"=→"IsAtHWLimit 2":bool)  [unwired: 1 in, 2 out]
          n107 = Wait (ms)(milliseconds to wait=u32 300) -> ()  [unwired: 1 out]
        }
        n108 = Wait (ms)(milliseconds to wait=u32 500) -> ()  [unwired: 1 out]
      }
    }
    frame #1 {
      w206 = FALSE
      n109 = disable-structure shown="Disabled" {
        frame Disabled {
          n110 = local read ".NET Refnum out 2"() -> (w207:refnum<k24>)
          n111 = local read ".NET Refnum out 1"() -> (w208:refnum<k24>)
          n112 = call "closeMotor.vi"(".NET Refnum in"=w208) -> ()  [unwired: 2 in]
          n113 = call "closeMotor.vi"(".NET Refnum in"=w207) -> ()  [unwired: 2 in]
        }
        frame Enabled {
        }
      }
      n114 = local write "Stop Button"(FALSE ("Stop Button")) -> ()
      n115 = property on="Iniciar" class="Bool (strict)"("DisabledEnum"=T1."Disabled and Grayed Out" ("Disabled")) -> ()  [unwired: 2 in, 2 out]
      n116 = local write "Motor 2"(w206) -> ()
      n117 = local write "Motor 1"(w206) -> ()
      "stop cronometro" <- TRUE ("stop cronometro")
    }
  }
